vi "IQ.vi"() -> ()   [LabVIEW 2022 SP3]
uses:
  <vilib>/Analysis/3filter.llb/Filter Passband Type.ctl
  <vilib>/Analysis/baseanly.llb/Mean (DBL).vi
  <vilib>/Analysis/2dsp.llb/Complex FFT.vi
  <vilib>/Analysis/3filter.llb/Butterworth Filter (DBL).vi
  <vilib>/gmath/NI_Gmath.lvlib
  <vilib>/Analysis/NI_AALPro.lvlib
  <vilib>/Analysis/NI_AALBase.lvlib
  <vilib>/Analysis/NI_AAL_SigProc.lvlib
panel:
  in  "Resp":bool
  in  "IQ":bool
  out "file":string
  in  "threshold y":dbl=25.0
  out "Resp Gate":bool[][](array[boolean])
  in  "Gate Length":i32=250
  in  "Gate Start":i32=-150
  out "Resp":dbl[][](array[numeric])
  in  "PRF":dbl=1.0
  out "All Resp":dbl[][](graph)
  out "Resp track":dbl[](graph)
  in  "AS Med Fil":i32=100
  in  "initial Skip index":i32=50
  out "Locations":dbl[][](array[numeric])
  in  "Use Selected Files":bool
  in  "Listbox":i32[](listbox)
  in  "file ext":string="*IQ*"
  in  "Choose Directory":path
  out "Q channel 4":dbl[][](graph)
  out "Q channel 2":dbl[][](graph)
  out "Q channel":dbl[][](graph)
  out "EKG 2":dbl[][](graph)
  out "data":i16[](array[numeric])
  out "EKG":dbl[][](graph)
  out "EKG":i16[][](graph)
  out "I  spectrogram":dbl[][](graph)
  out "Doppler Signal":dbl[][](graph)
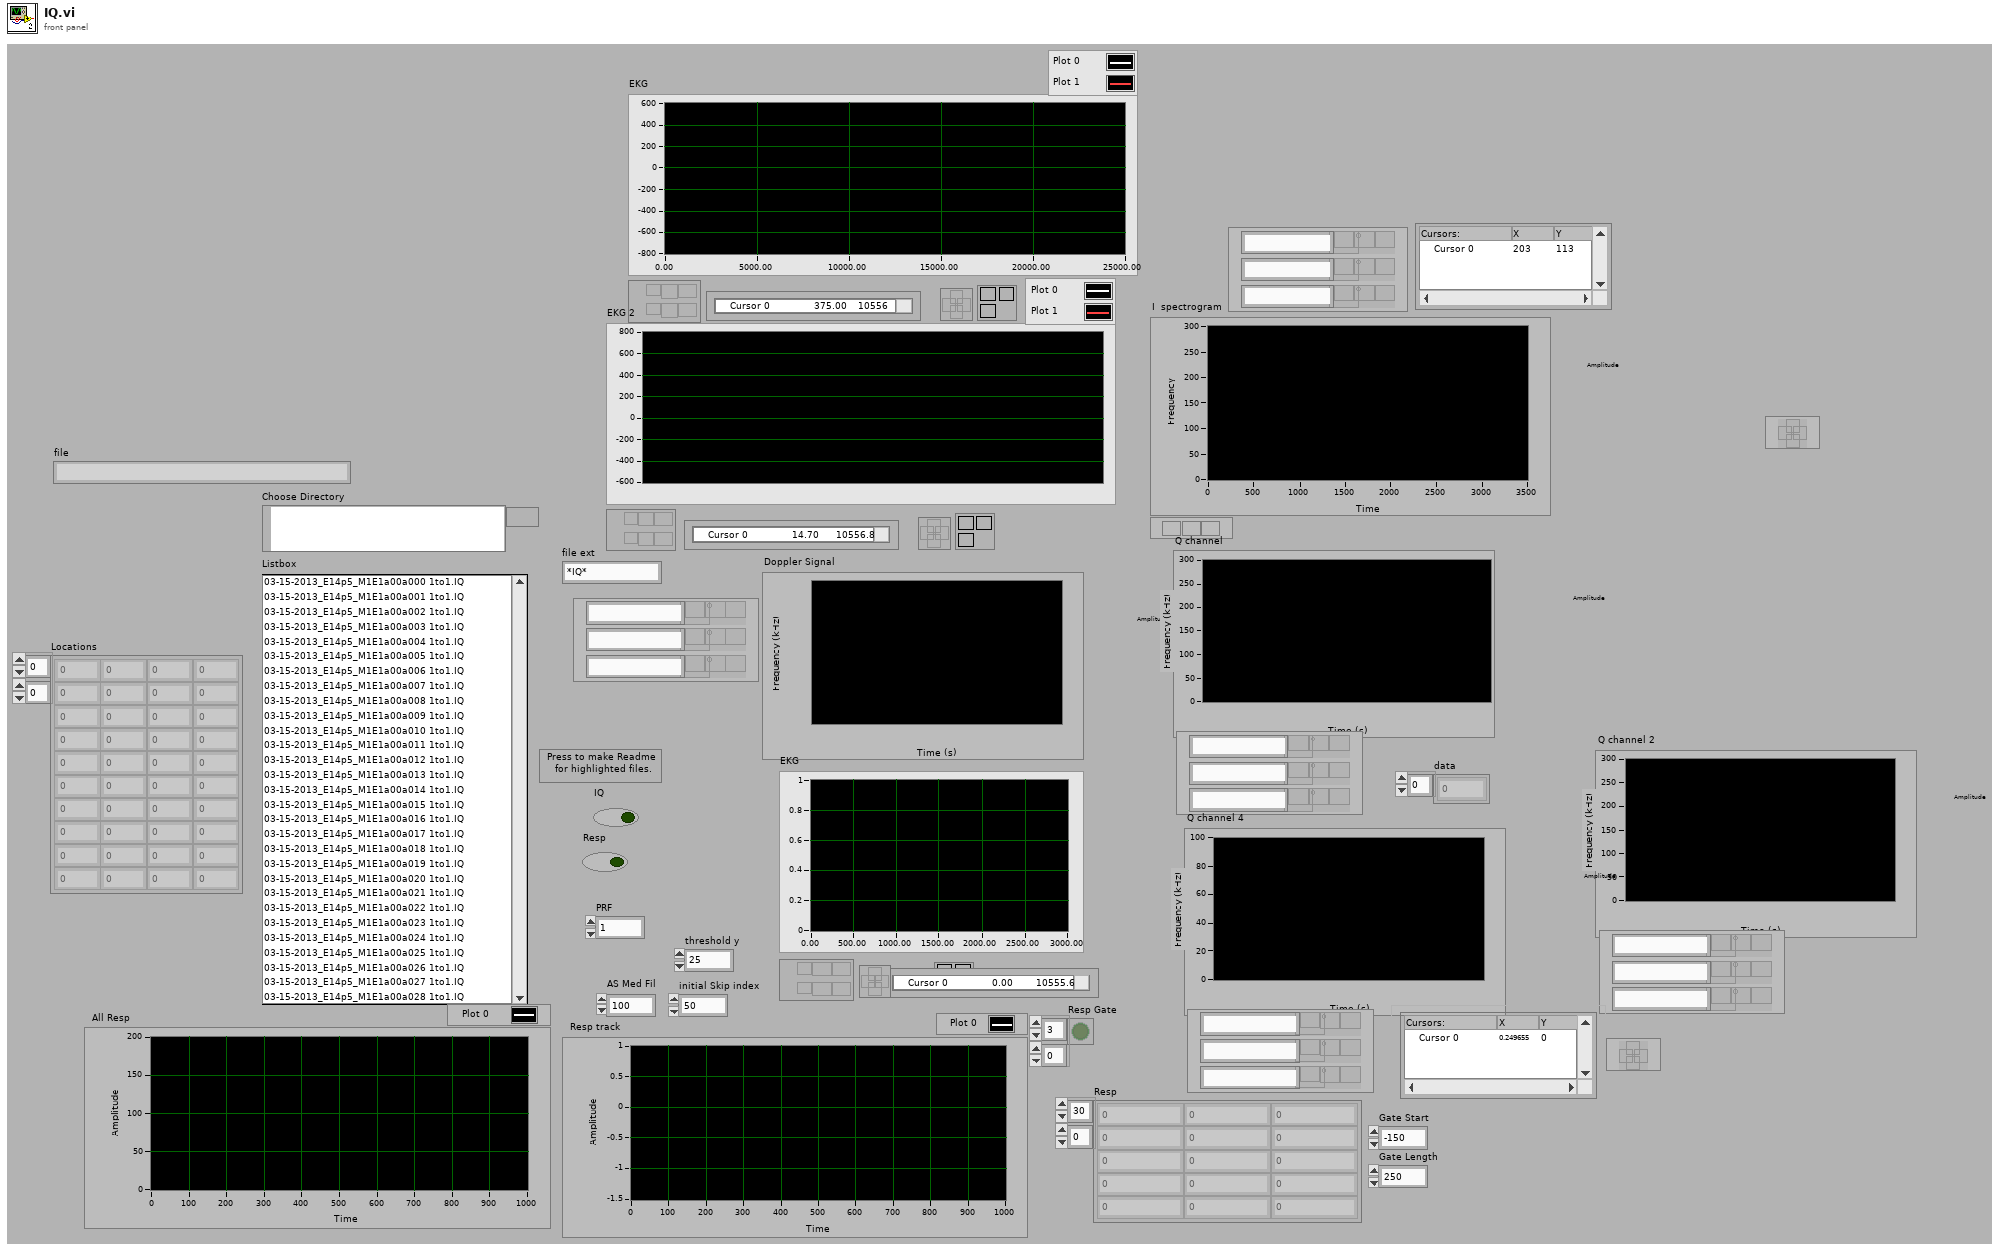
[diagram p1: front panel]
types:
  T1 = enum16{"big-endian, network order", "native, host order", "little-endian"}
  T2 = typedef "NI_AALBase.lvlib/Filter Passband Type.ctl" = enum32{"Lowpass", "Highpass", "Bandpass", "Bandstop"}
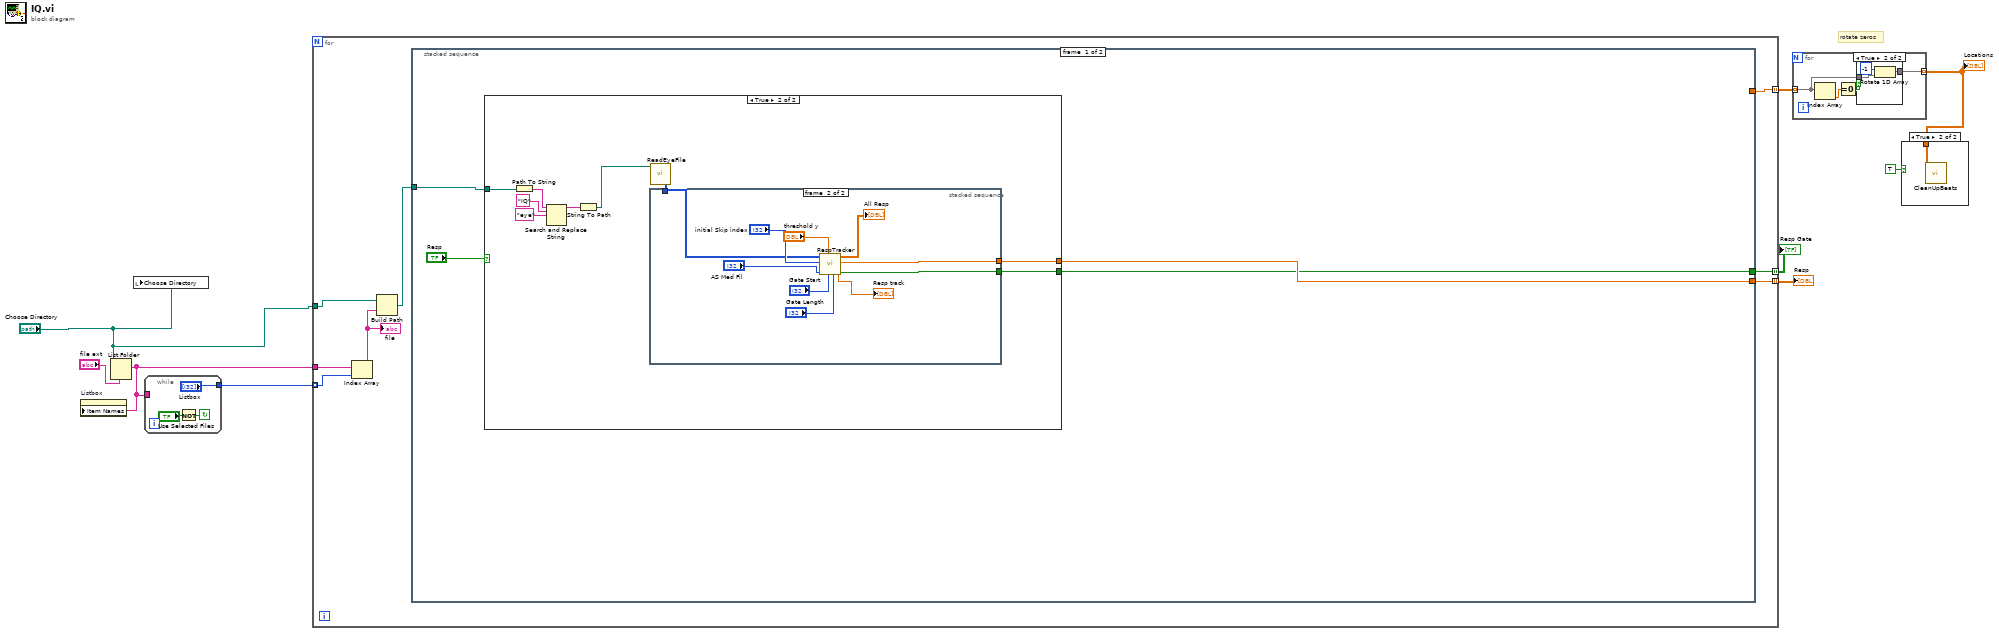
[diagram p0: block diagram]
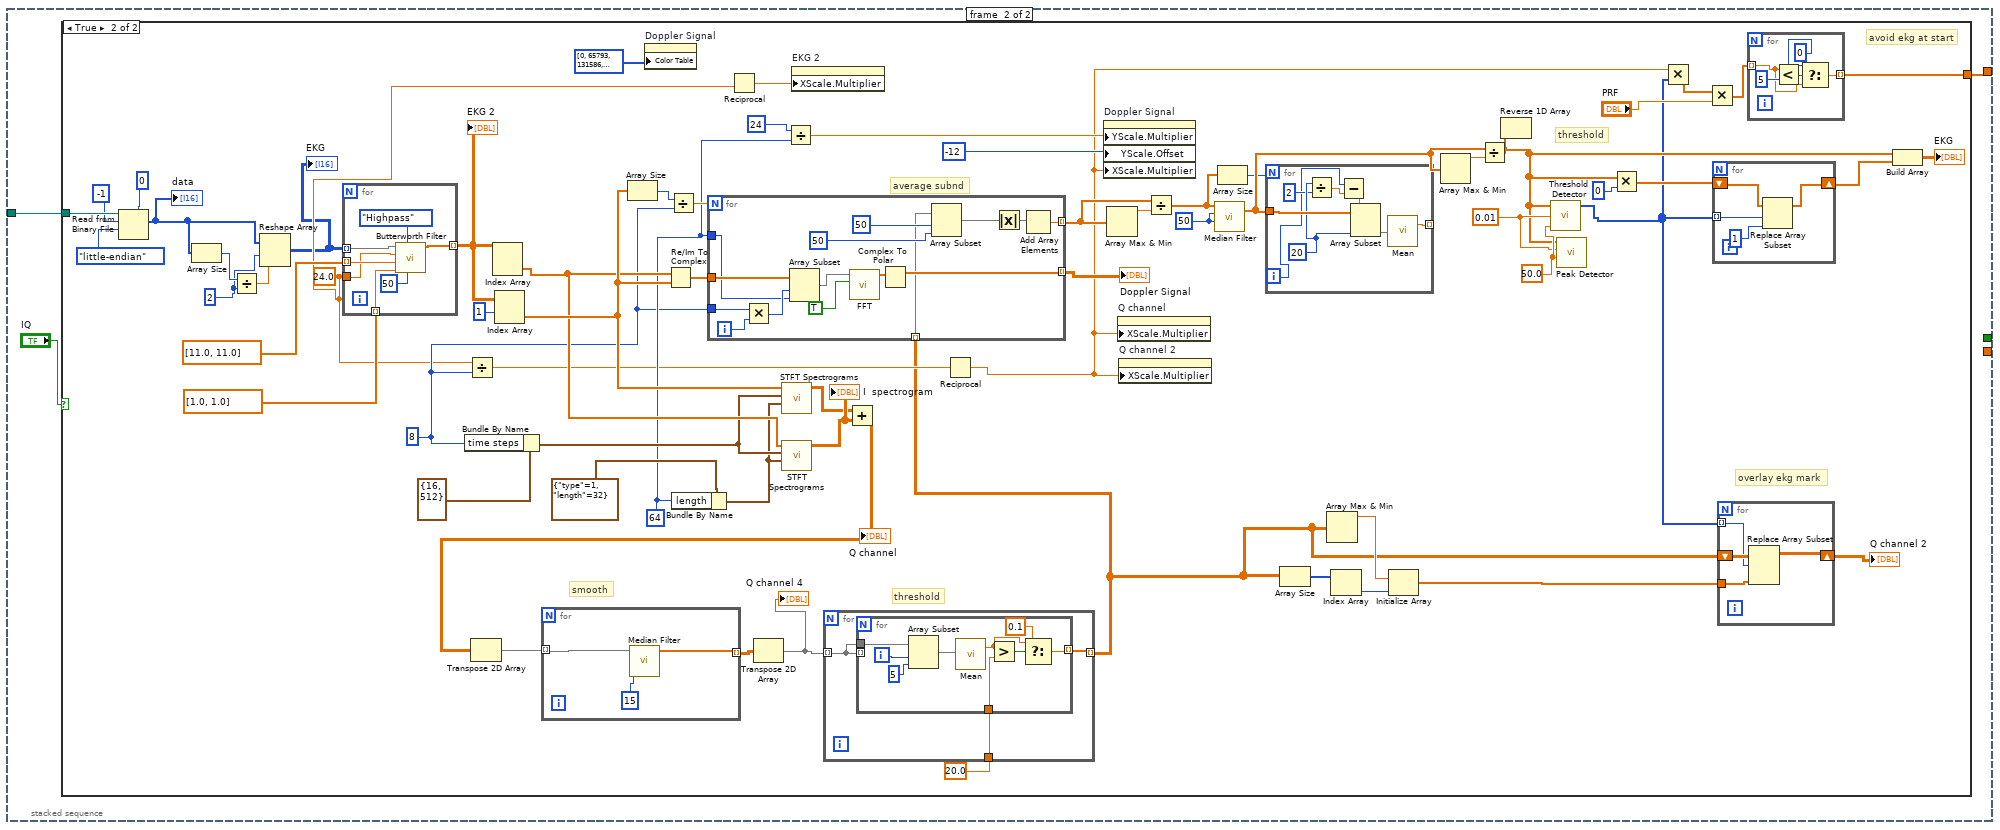
[diagram p6: hidden frame]
diagram:
  # "rotate zeros"
  n1 = List Folder(path="Choose Directory", pattern="file ext") -> (filenames=w7:string[])  [unwired: 1 in, 4 out]
  n2 = property on="Listbox" class="LstBox (strict)"("Item Names"=w7) -> ()  [unwired: 2 in, 2 out]
  n3 = local write "Choose Directory"("Choose Directory") -> ()
  n4 = while {
    tunnel: ["Listbox"] -> w8
    tunnel: w7 -> [_]
    stop <- w12 continue-if-true
    n5 = Not(x="Use Selected Files") -> (.not. x?=w12:bool)
  }
  n6 = for {
    tunnel: "Choose Directory" -> [w18]
    tunnel: w8 -> [w19] mode=indexing
    tunnel: w7 -> [w20]
    tunnel: [w15] -> w5 mode=indexing
    tunnel: [w14] -> w3 mode=indexing
    tunnel: [w13] -> w2 mode=indexing
    n7 = Index Array(array=w20, index=w19) -> (element=w17:string)
    "file" <- w17
    n8 = Build Path(base path=w18, name or relative path=w17) -> (appended path=w16:path)
    n9 = stacked-sequence {
      tunnel: w16 -> [w24 w46]
      tunnel: [_ w45] -> w15
      tunnel: [w23 _] -> w14
      tunnel: [w22 _] -> w13
      frame #0 {
        n10 = case shown="True" "Resp" {
          tunnel: w24 -> [_ w32]
          tunnel: [_ w28] -> w23
          tunnel: [_ w25] -> w22
          frame False {
          }
          frame True {
            n11 = Path To String(path=w32) -> (string=w33:string)
            n12 = Search and Replace String(input string=w33, search string="IQ", replace string="eye" ("replace string (\"\")")) -> (result string=w29:string)  [unwired: 5 in, 3 out]
            n13 = String To Path(string=w29) -> (path=w27:path)
            n14 = call "ReadEyeFile.vi"("new file path"=w27) -> ("2-D data array"=w26:i16[][])  [unwired: 1 in, 17 out]
            n15 = stacked-sequence {
              tunnel: [_ w39] -> w28
              tunnel: w26 -> [_ w36]
              tunnel: [_ w35] -> w25
              frame #0 {
              }
              frame #1 {
                n16 = call "RespTracker.vi"("Gate Length"="Gate Length", "Gate Start"="Gate Start", "threshold y"="threshold y", "AS Med Fil"="AS Med Fil", "initial Skip index"="initial Skip index", "2-D data array"=w36) -> ("Resp Gate"=w35:bool[], "RF Threshold"=→"Resp track":dbl[], "Locations"=w39:dbl[], "All curves"=→"All Resp":dbl[][])  [unwired: 2 in]
              }
            }
          }
        }
      }
      frame #1 {
        n17 = case shown="True" "IQ" {
          tunnel: w46 -> [_ w74]
          tunnel: [_ w56] -> w45
          frame False {
          }
          frame True {
            w70 = 50 ("left rank")
            w75 = 24.0 ("sampling freq: fs")
            w79 = 64 ("length")
            w78 = 8 ("time steps")
            w96 = 2
            w63 = 50.0 ("threshold")
            w62 = 0.01 ("threshold")
            # "avoid ekg at start"
            # "threshold"
            # "average subnd"
            # "threshold"
            # "smooth"
            # "overlay ekg mark"
            n18 = Read from Binary File(5:i16 0, 9:T1."little-endian" ("byte order (0:big-endian, network order)"), 10:-1 ("count (1)"), 11:w74) -> (2:w89:i16[])  [unwired: 2 in, 3 out]
            "data" <- w89
            n19 = Array Size(array=w89) -> (size(s)=w97:i32)
            n20 = Divide(x=w97, y=w96) -> (x/y=w95:dbl)
            n21 = Reshape Array(w89, w96, w95) -> (w48:i16[][])
            "EKG" <- w48
            n22 = for {
              tunnel: w48 -> [w146] mode=indexing
              tunnel: [w145] -> w47 mode=indexing
              tunnel: dbl[] [11.0, 11.0] -> [w142] mode=indexing
              tunnel: dbl[] [1.0, 1.0] -> [w141] mode=indexing
              tunnel: w75 -> [w140]
              n23 = call-poly <vilib>:"Butterworth Filter.vi"("order"=50, "filter type"=Filter_Passband_Type."Highpass", "low cutoff freq: fl"=w141, "high cutoff freq: fh"=w142, "sampling freq: fs"=w140, "X"=w146) -> ("Filtered X"=w145:dbl[])  [unwired: 2 in, 1 out]
            }
            "EKG 2" <- w47
            n24 = Bundle By Name(cluster=cluster{"time steps":i32, "frequency bins":i32} {"time steps"=16, "frequency bins"=512} ("time-freq sampling info"), "time steps"=w78) -> (w82:cluster{"time steps":i32, "frequency bins":i32})
            n25 = Divide(x=w75, y=w78) -> (x/y=w76:dbl)
            n26 = Index Array(array=w47) -> (element=w90:dbl[])  [unwired: 2 in]
            n27 = Index Array(array=w47, index (row)=1) -> (element=w109:dbl[])  [unwired: 1 in]
            n28 = Array Size(array=w109) -> (size(s)=w110:i32)
            n29 = property on="Doppler Signal" class="IntGraph (strict)"("Color Table"=u32[] [0, 65793, 131586, 197379, 263172, 328965, 394758, 460551, 526344, 592137, 657930, 723723, 789516, 855309, 921102, 986895, 1052688, 1118481, 1184274, 1250067, 1315860, 1381653, 1447446, 1513239, 1579032, 1644825, 1710618, 1776411, 1842204, 1907997, 1973790, 2039583, 2105376, 2171169, 2236962, 2302755, 2368548, 2434341, 2500134, 2565927, 2631720, 2697513, 2763306, 2829099, 2894892, 2960685, 3026478, 3092271, 3158064, 3223857, 3289650, 3355443, 3421236, 3487029, 3552822, 3618615, 3684408, 3750201, 3815994, 3881787, 3947580, 4013373, 4079166, 4144959, 4210752, 4276545, 4342338, 4408131, 4473924, 4539717, 4605510, 4671303, 4737096, 4802889, 4868682, 4934475, 5000268, 5066061, 5131854, 5197647, 5263440, 5329233, 5395026, 5460819, 5526612, 5592405, 5658198, 5723991, 5789784, 5855577, 5921370, 5987163, 6052956, 6118749, 6184542, 6250335, 6316128, 6381921, 6447714, 6513507, 6579300, 6645093, 6710886, 6776679, 6842472, 6908265, 6974058, 7039851, 7105644, 7171437, 7237230, 7303023, 7368816, 7434609, 7500402, 7566195, 7631988, 7697781, 7763574, 7829367, 7895160, 7960953, 8026746, 8092539, 8158332, 8224125, 8289918, 8355711, 8421504, 8487297, 8553090, 8618883, 8684676, 8750469, 8816262, 8882055, 8947848, 9013641, 9079434, 9145227, 9211020, 9276813, 9342606, 9408399, 9474192, 9539985, 9605778, 9671571, 9737364, 9803157, 9868950, 9934743, 10000536, 10066329, 10132122, 10197915, 10263708, 10329501, 10395294, 10461087, 10526880, 10592673, 10658466, 10724259, 10790052, 10855845, 10921638, 10987431, 11053224, 11119017, 11184810, 11250603, 11316396, 11382189, 11447982, 11513775, 11579568, 11645361, 11711154, 11776947, 11842740, 11908533, 11974326, 12040119, 12105912, 12171705, 12237498, 12303291, 12369084, 12434877, 12500670, 12566463, 12632256, 12698049, 12763842, 12829635, 12895428, 12961221, 13027014, 13092807, 13158600, 13224393, 13290186, 13355979, 13421772, 13487565, 13553358, 13619151, 13684944, 13750737, 13816530, 13882323, 13948116, 14013909, 14079702, 14145495, 14211288, 14277081, 14342874, 14408667, 14474460, 14540253, 14606046, 14671839, 14737632, 14803425, 14869218, 14935011, 15000804, 15066597, 15132390, 15198183, 15263976, 15329769, 15395562, 15461355, 15527148, 15592941, 15658734, 15724527, 15790320, 15856113, 15921906, 15987699, 16053492, 16119285, 16185078, 16250871, 16316664, 16382457, 16448250, 16514043, 16579836, 16645629, 16711422, 16711680]) -> ()  [unwired: 2 in, 2 out]
            n30 = Re/Im To Complex(1:w109, 2:w90) -> (0:w93:cdb[])
            n31 = Divide(x=w110, y=w78) -> (x/y=w107:dbl)
            n32 = Bundle By Name(cluster=cluster{"type":u32, "length":i32} {"type"=1, "length"=32} ("window info"), "length"=w79) -> (w80:cluster{"type":u32, "length":i32})
            n33 = Reciprocal(x=w75) -> (1/x=w77:dbl)
            n34 = call <vilib>:"STFT Spectrograms.vi"("window info"=w80, "time-freq sampling info"=w82, "X"=w109) -> ("STFT Spectrogram {X}"=w68:dbl[][])  [unwired: 7 in, 1 out]
            n35 = call <vilib>:"STFT Spectrograms.vi"("window info"=w80, "time-freq sampling info"=w82, "X"=w90) -> ("STFT Spectrogram {X}"=w69:dbl[][])  [unwired: 7 in, 1 out]
            "I  spectrogram" <- w69
            n36 = Divide(x=24, y=w79) -> (x/y=w104:dbl)
            n37 = property on="EKG 2" class="WFGraph (strict)"("XScale.Multiplier"=w77) -> ()  [unwired: 2 in, 2 out]
            n38 = Add(x=w68, y=w69) -> (x+y=w54:dbl[][])
            "Q channel" <- w54
            n39 = Transpose 2D Array(2D array=w54) -> (transposed array=w60:dbl[][])
            n40 = for {
              tunnel: w60 -> [w114] mode=indexing
              tunnel: [w113] -> w61 mode=indexing
              w112 = 15 ("left rank")
              n41 = call <vilib>:"Median Filter.vi"("right rank"=w112, "left rank"=w112, "X"=w114) -> ("Filtered X"=w113:dbl[])  [unwired: 7 in, 1 out]
            }
            n42 = Transpose 2D Array(2D array=w61) -> (transposed array=w53:dbl[][])
            "Q channel 4" <- w53
            n43 = for {
              tunnel: w53 -> [w125] mode=indexing
              tunnel: 20.0 ("y") -> [w126]
              tunnel: [w124] -> w55 mode=indexing
              n44 = for {
                tunnel: w125 -> [_] mode=indexing
                tunnel: w125 -> [w135]
                tunnel: w126 -> [w129]
                tunnel: [w130] -> w124 mode=indexing
                i -> [w134]
                n45 = Array Subset(array=w135, index=w134, length=5) -> (w132:dbl[])
                n46 = call-poly <vilib>:"Mean.vi"("X"=w132) -> ("mean"=w127:dbl)  [unwired: 1 out]
                n47 = Greater?(x=w127, y=w129) -> (0:w131:bool)
                n48 = Select(t=w127, s=w131, f=0.1) -> (s? t:f=w130:dbl)
              }
            }
            n49 = for {
              N: w107 -> [_]
              tunnel: w93 -> [w169]
              tunnel: w79 -> [w158]
              tunnel: w78 -> [w167]
              tunnel: [w156] -> w94 mode=indexing
              tunnel: [w161] -> w102 mode=indexing
              tunnel: w55 -> [w155] mode=indexing
              i -> [w168]
              n50 = Multiply(x=w167, y=w168) -> (x*y=w166:i32)
              n51 = Array Subset(array=w169, index=w166, length=w158) -> (w165:cdb[])
              n52 = call-poly <vilib>:"FFT.vi"("shift?"=TRUE, "X"=w165) -> ("FFT {X}"=w163:cdb[])  [unwired: 8 in, 1 out]
              n53 = Complex To Polar(r * e^(i*theta)=w163) -> (r=w156:dbl[])  [unwired: 1 out]
              n54 = Array Subset(array=w155, index=50, length=50) -> (w160:dbl[])
              n55 = Absolute Value(x=w160) -> (abs(x)=w162:dbl[])
              n56 = Add Array Elements(numeric array=w162) -> (sum=w161:dbl)
            }
            "Doppler Signal" <- w94
            n57 = Reciprocal(x=w76) -> (1/x=w66:dbl)
            n58 = property on="Doppler Signal" class="IntGraph (strict)"("YScale.Multiplier"=w104, "YScale.Offset"=-12, "XScale.Multiplier"=w66) -> ()  [unwired: 2 in, 2 out]
            n59 = Array Max & Min(array=w102) -> (max value=w103:dbl)  [unwired: 3 out]
            n60 = property on="Q channel" class="IntGraph (strict)"("XScale.Multiplier"=w66) -> ()  [unwired: 2 in, 2 out]
            n61 = property on="Q channel 2" class="IntGraph (strict)"("XScale.Multiplier"=w66) -> ()  [unwired: 2 in, 2 out]
            n62 = Divide(x=w102, y=w103) -> (x/y=w65:dbl[])
            n63 = call <vilib>:"Median Filter.vi"("right rank"=w70, "left rank"=w70, "X"=w65) -> ("Filtered X"=w67:dbl[])  [unwired: 7 in, 1 out]
            n64 = Array Size(array=w65) -> (size(s)=w51:i32)
            n65 = for {
              N: w51 -> [_]
              tunnel: w67 -> [w154]
              tunnel: [w152] -> _ mode=indexing
              i -> [w147]
              w151 = 20
              n66 = Divide(x=w151, y=2) -> (x/y=w149:dbl)
              n67 = Subtract(x=w147, y=w149) -> (x-y=w148:dbl)
              n68 = Array Subset(array=w154, index=w148, length=w151) -> (w153:dbl[])
              n69 = call-poly <vilib>:"Mean.vi"("X"=w153) -> ("mean"=w152:dbl)  [unwired: 1 out]
            }
            n70 = Array Size(array=w55) -> (size(s)=w88:i32[])
            n71 = Array Max & Min(array=w55) -> (max value=w86:dbl)  [unwired: 3 out]
            n72 = Index Array(array=w88) -> (element=w87:i32)  [unwired: 1 in]
            n73 = Initialize Array(w86, w87) -> (w85:dbl[])
            n74 = Array Max & Min(array=w67) -> (max value=w101:dbl)  [unwired: 3 out]
            n75 = Divide(x=w67, y=w101) -> (x/y=w50:dbl[])
            n76 = Reverse 1D Array(array=w50) -> ()  [unwired: 1 out]
            n77 = call <vilib>:"Threshold Detector.vi"("width"=w63, "threshold"=w62, "X"=w50) -> ("Indices"=w49:i32[])  [unwired: 2 out]
            n78 = call <vilib>:"Peak Detector.vi"("width"=w63, "threshold"=w62, "X"=w50) -> ()  [unwired: 4 in, 5 out]
            n79 = Multiply(x=w50, y=0) -> (x*y=w99:dbl[])
            n80 = Multiply(x=w66, y=w49) -> (x*y=w58:dbl[])
            n81 = Multiply(x=w58, y="PRF") -> (x*y=w57:dbl[])
            n82 = for {
              tunnel: w49 -> [w136] mode=indexing
              shift-right: [w137] -> w98
              shift-left: w99 -> [w139]
              n83 = Replace Array Subset(array=w139, new element=1, index=w136) -> (w137:dbl[])
            }
            n84 = for {
              tunnel: w49 -> [w121] mode=indexing
              tunnel: w85 -> [w122]
              shift-right: [w120] -> w84
              shift-left: w55 -> [w123]
              n85 = Replace Array Subset(array=w123, new element=w122, index (row)=w121) -> (w120:dbl[][])  [unwired: 1 in]
            }
            "Q channel 2" <- w84
            n86 = for {
              tunnel: w57 -> [w117] mode=indexing
              tunnel: [w116] -> w56 mode=indexing
              n87 = Less?(x=w117, y=5) -> (x < y?=w118:bool)
              n88 = Select(t=0 ("y"), s=w118, f=w117) -> (s? t:f=w116:dbl)
            }
            n89 = Build Array(w50, w98) -> (→"EKG":dbl[][])
          }
        }
      }
    }
  }
  "Resp" <- w3
  "Resp Gate" <- w2
  n90 = for {
    tunnel: w5 -> [w171] mode=indexing
    tunnel: [w170] -> w4 mode=indexing
    n91 = Index Array(array=w171) -> (element=w173:dbl)  [unwired: 1 in]
    n92 = Equal To 0?(x=w173) -> (x = 0?=w172:bool)
    n93 = case shown="True" w172 {
      tunnel: w171 -> [w174 w177]
      tunnel: [w174 w176] -> w170
      frame False {
      }
      frame True {
        n94 = Rotate 1D Array(1:w177, 2:-1 ("n")) -> (0:w176:dbl[])
      }
    }
  }
  "Locations" <- w4
  n95 = case shown="True" TRUE {
    tunnel: w4 -> [_ w178]
    frame False {
    }
    frame True {
      n96 = call "CleanUpBeats.vi"("Beat INput"=w178) -> ()  [unwired: 9 in, 2 out]
    }
  }
